vi "PYTHON Symple Execute.vi"() -> ()   [LabVIEW 2009]
uses:
  library/PYTHON Get Float Data.vi
  library/PYTHON Get String Data.vi
  library/PYTHON Set Integer Data.vi
  library/PYTHON Set Float Data.vi
  library/PYTHON Set String Data.vi
panel:
  out "types":string[](array[string])
  out "names":string[](array[string])
  out "error out":errorcluster
  in  "error in (no error)":errorcluster
  in  "script":string="x = \"Python\"\ny = \"cool\"\nz = \"!\"*len(x)\nresult=\"%s%s is %s%s\"%(text,x,y,z)\nout = 2*val/div\nnum = out*val/len(x)"
  out "out (really a float)":string
  in  "div":i32=9
  out "num":dbl format="%.6f"
  out "result":string
  in  "Text":string="Hello brave World!\r"
  in  "val":dbl=4.0 format="%.2f"
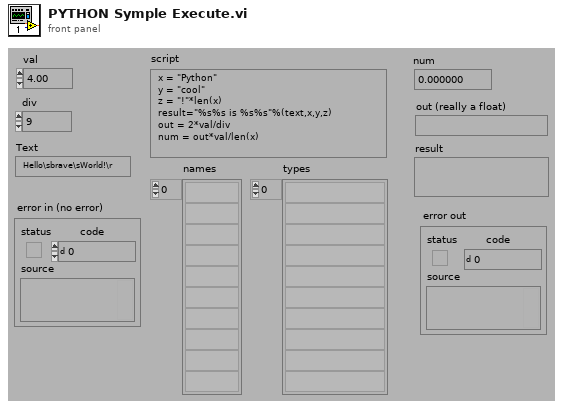
[diagram p1: front panel]
types:
  T1 = typedef "PYTHON Session Refnum.ctl" = refnum<k1>
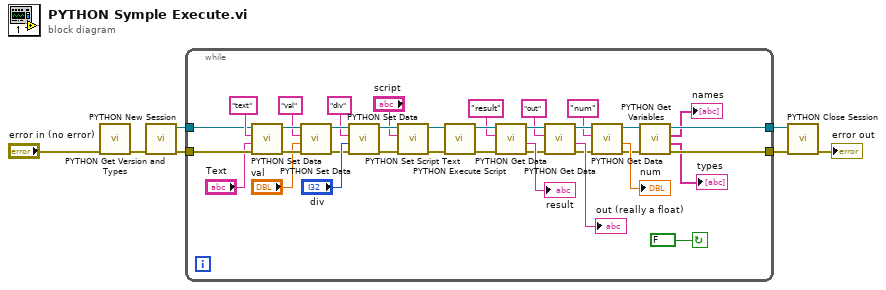
[diagram p0: block diagram]
diagram:
  n1 = call "PYTHON Get Version and Types.vi"("error in (no error)"="error in (no error)") -> ("error out"=w5:errorcluster)  [unwired: 4 in, 2 out]
  n2 = call "PYTHON New Session.vi"("error in (no error)"=w5) -> ("error out"=w7:errorcluster, "Python Session"=w6:T1)  [unwired: 5 in]
  n3 = while {
    tunnel: w7 -> [w43]
    tunnel: w6 -> [w40]
    tunnel: [w10] -> w4
    tunnel: [w11] -> w3
    stop <- FALSE continue-if-true
    n4 = call-poly "PYTHON Set Data.vi"("error in (no error)"=w43, "value"="Text", "variable name"="text", "Python Session in"=w40) -> ("error out"=w39:errorcluster, "Python Session out"=w38:T1)  [unwired: 2 in]
    n5 = call-poly "PYTHON Set Data.vi"("error in (no error)"=w39, "value"="val", "variable name"="val", "Python Session in"=w38) -> ("error out"=w35:errorcluster, "Python Session out"=w34:T1)  [unwired: 2 in]
    n6 = call-poly "PYTHON Set Data.vi"("error in (no error)"=w35, "value"="div", "variable name"="div", "Python Session in"=w34) -> ("error out"=w30:errorcluster, "Python Session out"=w31:T1)  [unwired: 2 in]
    n7 = call "PYTHON Set Script Text.vi"("error in (no error)"=w30, "script text"="script", "Python Session in"=w31) -> ("error out"=w27:errorcluster, "Python Session out"=w28:T1)  [unwired: 3 in]
    n8 = call "PYTHON Execute Script.vi"("error in (no error)"=w27, "Python Session in"=w28) -> ("error out"=w25:errorcluster, "Python Session out"=w26:T1)  [unwired: 4 in]
    n9 = call-poly "PYTHON Get Data.vi"("error in (no error)"=w25, "variable name"="result", "Python Session in"=w26) -> ("error out"=w20:errorcluster, "value"=→"result":string, "Python Session out"=w21:T1)  [unwired: 2 in]
    n10 = call-poly "PYTHON Get Data.vi"("error in (no error)"=w20, "variable name"="out", "Python Session in"=w21) -> ("error out"=w18:errorcluster, "value"=→"out (really a float)":string, "Python Session out"=w19:T1)  [unwired: 2 in]
    n11 = call-poly "PYTHON Get Data.vi"("error in (no error)"=w18, "variable name"="num", "Python Session in"=w19) -> ("error out"=w13:errorcluster, "value"=→"num":dbl, "Python Session out"=w12:T1)  [unwired: 2 in]
    n12 = call "PYTHON Get Variables.vi"("error in (no error)"=w13, "Python Session in"=w12) -> ("error out"=w10:errorcluster, "types"=→"types":string[], "names"=→"names":string[], "Python Session out"=w11:T1)  [unwired: 2 in]
  }
  n13 = call "PYTHON Close Session.vi"("error in (no error)"=w4, "Python Session in"=w3) -> ("error out"=→"error out":errorcluster)  [unwired: 5 in]
